vi "Apply Dichotomie on Coordinates.vi"(4 "Dichotomie in":i32, 6 "Time factor in":dbl format="%#_13g", 10 "Movable in":refnum<class "Movable.lvclass">) -> (2 "Coordinates with dichotomie[]":T1[](array[typedef]), 5 "Dichotomie out":i32=10)   [LabVIEW 2021, in "Game Board.lvclass"]
doc: "MIT Licence\nCopyright (c) 2024 David Grollier"
uses:
  Game Board.lvclass
  Type Def/Coordinates.ctl
  Game Board Component/Movable/Movable.lvclass
  C:/Users/David/Documents/GameSoccerSpace/Source/Game Componants/Game Componants.lvclass
  Game Board Component/Movable/Movable.lvclass/Movable.ctl
  Game Componants.lvclass/Game Componants.ctl
  Game Componants.lvclass
panel:
  out "test":T1[](array[typedef])
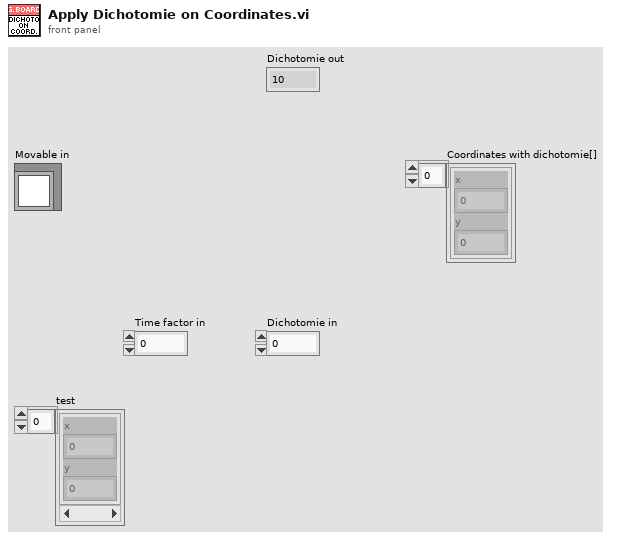
[diagram p1: front panel]
types:
  T1 = typedef "Coordinates.ctl" = cluster{"x":dbl, "y":dbl}
  T2 = typedef "Velocity.ctl" = cluster{"Vx":dbl, "Vy":dbl}
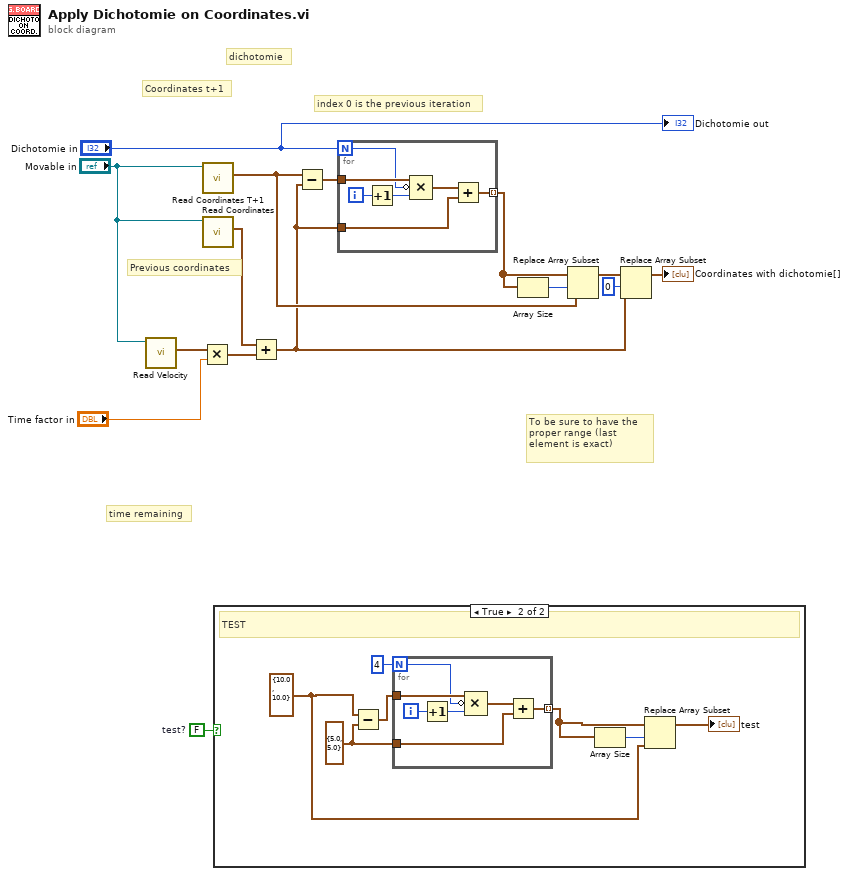
[diagram p0: block diagram]
diagram:
  w7 = FALSE  # test?
  # "time remaining"
  # "Coordinates t+1"
  # "Previous coordinates"
  # "To be sure to have the proper range (last element is exact)"
  # "index 0 is the previous iteration"
  # "dichotomie"
  n1 = call-dynamic "Read Velocity.vi"("Movable in"="Movable in") -> ("Velocity"=w5:T2)  [unwired: 10 in]
  n2 = Multiply(x=w5, y="Time factor in") -> (x*y=w2:T2)
  n3 = call "Read Coordinates T+1.vi"("Movable in"="Movable in") -> ("Coordinates"=w12:T1)  [unwired: 10 in]
  n4 = call "Read Coordinates.vi"("Game Componants in"="Movable in") -> ("Coordinates"=w3:T1)  [unwired: 10 in]
  n5 = case shown="True" w7 {
    frame False {
    }
    frame True {
      w19 = T1 {"x"=5.0, "y"=5.0} ("Coordinates")
      w20 = T1 {"x"=10.0, "y"=10.0} ("Coordinates")
      # "TEST"
      n6 = Subtract(x=w20, y=w19) -> (x-y=w18:T1)
      n7 = for {
        N: 4 -> [w28]
        tunnel: w18 -> [w29]
        tunnel: [w25] -> w22 mode=indexing
        tunnel: w19 -> [w23]
        i -> [w26]
        n8 = Increment(x=w26) -> (x+1=w24:i32)
        n9 = Compound Arithmetic op=MULTIPLY(w29, invert w28, w24) -> (w27:T1)
        n10 = Add(x=w27, y=w23) -> (x+y=w25:T1)
      }
      n11 = Array Size(array=w22) -> (size(s)=w21:i32)
      n12 = Replace Array Subset(array=w22, new element=w20, index=w21) -> (→"test":T1[])
    }
  }
  n13 = Add(x=w3, y=w2) -> (x+y=w1:T1)
  n14 = Subtract(x=w12, y=w1) -> (x-y=w15:T1)
  n15 = for {
    N: "Dichotomie in" -> [w35]
    tunnel: w15 -> [w36]
    tunnel: [w32] -> w13 mode=indexing
    tunnel: w1 -> [w30]
    i -> [w33]
    n16 = Increment(x=w33) -> (x+1=w31:i32)
    n17 = Compound Arithmetic op=MULTIPLY(w36, invert w35, w31) -> (w34:T1)
    n18 = Add(x=w34, y=w30) -> (x+y=w32:T1)
  }
  n19 = Array Size(array=w13) -> (size(s)=w14:i32)
  n20 = Replace Array Subset(array=w13, new element=w12, index=w14) -> (w11:T1[])
  n21 = Replace Array Subset(array=w11, new element=w1, index=0) -> (→"Coordinates with dichotomie[]":T1[])
  "Dichotomie out" <- "Dichotomie in"
